vi "LSX Connect Ex.vi"(8 "error in (no error)":errorcluster, 10 "pAControlInitPar":T1, 11 "lLSID":i32) -> (0 "error out":errorcluster, 2 "pAControlInitPar out":T1, 3 "function return":i32)   [LabVIEW 2018, in "Tango.lvlib"]
doc: "TANGOAPI int TANGOCALL LSX_ConnectEx (int lLSID, TLS_ControlInitPar *pAControlInitPar);"
uses:
  Tango.lvlib
  SubVIs/Tango_DLL.dll
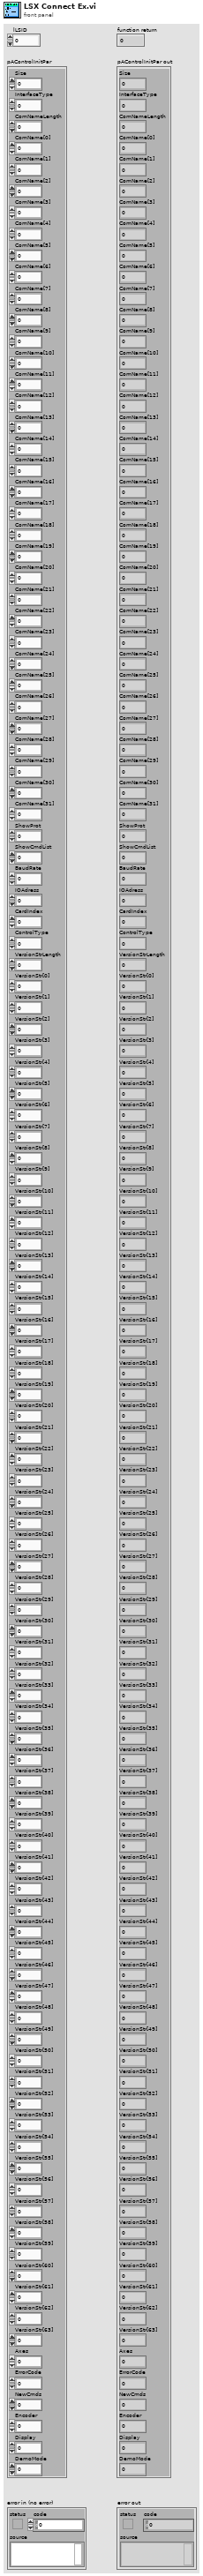
[diagram p1: front panel]
types:
  T1 = cluster{"Size":i32, "InterfaceType":i32, "ComNameLength":i8, "ComName[0]":i8, "ComName[1]":i8, "ComName[2]":i8, "ComName[3]":i8, "ComName[4]":i8, "ComName[5]":i8, "ComName[6]":i8, "ComName[7]":i8, "ComName[8]":i8, "ComName[9]":i8, "ComName[10]":i8, "ComName[11]":i8, "ComName[12]":i8, "ComName[13]":i8, "ComName[14]":i8, "ComName[15]":i8, "ComName[16]":i8, "ComName[17]":i8, "ComName[18]":i8, "ComName[19]":i8, "ComName[20]":i8, "ComName[21]":i8, "ComName[22]":i8, "ComName[23]":i8, "ComName[24]":i8, "ComName[25]":i8, "ComName[26]":i8, "ComName[27]":i8, "ComName[28]":i8, "ComName[29]":i8, "ComName[30]":i8, "ComName[31]":i8, "ShowProt":i32, "ShowCmdList":i32, "BaudRate":i32, "IOAdress":i32, "CardIndex":i32, "ControlType":i32, "VersionStrLength":i8, "VersionStr[0]":i8, "VersionStr[1]":i8, "VersionStr[2]":i8, "VersionStr[3]":i8, "VersionStr[4]":i8, "VersionStr[5]":i8, "VersionStr[6]":i8, "VersionStr[7]":i8, "VersionStr[8]":i8, "VersionStr[9]":i8, "VersionStr[10]":i8, "VersionStr[11]":i8, "VersionStr[12]":i8, "VersionStr[13]":i8, "VersionStr[14]":i8, "VersionStr[15]":i8, "VersionStr[16]":i8, "VersionStr[17]":i8, "VersionStr[18]":i8, "VersionStr[19]":i8, "VersionStr[20]":i8, "VersionStr[21]":i8, "VersionStr[22]":i8, "VersionStr[23]":i8, "VersionStr[24]":i8, "VersionStr[25]":i8, "VersionStr[26]":i8, "VersionStr[27]":i8, "VersionStr[28]":i8, "VersionStr[29]":i8, "VersionStr[30]":i8, "VersionStr[31]":i8, "VersionStr[32]":i8, "VersionStr[33]":i8, "VersionStr[34]":i8, "VersionStr[35]":i8, "VersionStr[36]":i8, "VersionStr[37]":i8, "VersionStr[38]":i8, "VersionStr[39]":i8, "VersionStr[40]":i8, "VersionStr[41]":i8, "VersionStr[42]":i8, "VersionStr[43]":i8, "VersionStr[44]":i8, "VersionStr[45]":i8, "VersionStr[46]":i8, "VersionStr[47]":i8, "VersionStr[48]":i8, "VersionStr[49]":i8, "VersionStr[50]":i8, "VersionStr[51]":i8, "VersionStr[52]":i8, "VersionStr[53]":i8, "VersionStr[54]":i8, "VersionStr[55]":i8, "VersionStr[56]":i8, "VersionStr[57]":i8, "VersionStr[58]":i8, "VersionStr[59]":i8, "VersionStr[60]":i8, "VersionStr[61]":i8, "VersionStr[62]":i8, "VersionStr[63]":i8, "Axes":i32, "ErrorCode":i32, "NewCmds":i32, "Encoder":i32, "Display":i32, "DemoMode":i32}
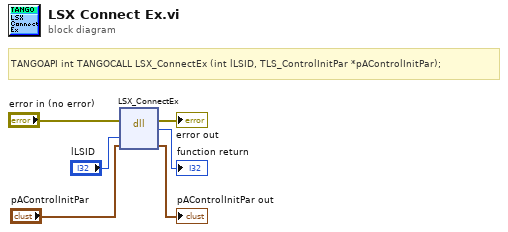
[diagram p0: block diagram]
diagram:
  # "TANGOAPI int TANGOCALL LSX_ConnectEx (int lLSID, TLS_ControlInitPar *pAControlInitPar);"
  n1 = dll-call lib="C:/Users/Familie/Documents/LabviewIX81/lib/TANGO Stage/SubVIs/Tango_DLL.*" fn="LSX_ConnectEx"(error in="error in (no error)", "lLSID"="lLSID", "pAControlInitPar"="pAControlInitPar") -> (error out=→"error out":errorcluster, →"function return":i32, "pAControlInitPar"=→"pAControlInitPar out":T1)  [unwired: 3 in, 1 out]
